vi "AxisGetConfFromFile.vi"(7 "conf file path":path caption="selected path", 8 "error in (no error)":errorcluster, 10 "AxisWriteValuesIn":T3={"AxisTarget"=0.0, "AxisTargetVel"=1.0, "AxisStartReq"=FALSE, "AxisStopReq"=FALSE, "AxisClearReq"=FALSE, "AxisMovetype"=FALSE, "AxisMotorON"=FALSE, "MoveModeControl"=4, "AxisHomingVel"=1.0, "AxisAccDecc"=30.0} {"MoveModeControl" items=["Absolute", "Relative", "Velocity", "Homing"]}, 11 "AxisConfigurationIn":T4={"AxisHomeType"=1, "AxisBacklash"=0.0, "AxisGain"=1.0, "AxisOffset"=0.0, "AxisUnit"=1, "ReqConfRead"=FALSE, "ReqConfWrite"=FALSE, "AxisName"="", "AxisAccDecc"=0.0, "AxisHomeVel"=0.0} {"AxisUnit" items=["mm", "°"]; "AxisHomeType" items=["no homing"=0, "forward limit switch"=1, "backward limit switch"=2, "forward reference"=4, "backward reference"=8]}) -> (0 "error out":errorcluster, 1 "AditionalConfigOut":T2 {"UnitsControl" items=["mm", "°"]}, 2 "AxisWriteValuesOut":T3={"AxisTarget"=0.0, "AxisTargetVel"=1.0, "AxisStartReq"=FALSE, "AxisStopReq"=FALSE, "AxisClearReq"=FALSE, "AxisMovetype"=FALSE, "AxisMotorON"=FALSE, "MoveModeControl"=4, "AxisHomingVel"=1.0, "AxisAccDecc"=30.0} {"MoveModeControl" items=["Absolute", "Relative", "Velocity", "Homing"]}, 3 "AxisConfigurationOut":T4={"AxisHomeType"=1, "AxisBacklash"=0.0, "AxisGain"=1.0, "AxisOffset"=0.0, "AxisUnit"=1, "ReqConfRead"=FALSE, "ReqConfWrite"=FALSE, "AxisName"="", "AxisAccDecc"=0.0, "AxisHomeVel"=0.0} {"AxisUnit" items=["mm", "°"]; "AxisHomeType" items=["no homing"=0, "forward limit switch"=1, "backward limit switch"=2, "forward reference"=4, "backward reference"=8]}, 4 "Comunication":T1={"DeviceIDCtrl"=1, "ProtocolCtrl"=enum."Modbus RTU", "COMportCtrl"="", "IPCtrl"=""})   [LabVIEW 2020, in "SMCD14_lib.lvlib"]
uses:
  SMCD14_lib.lvlib
  AxisConfiguration_typedef.ctl
  AxisWriteValues_typedef.ctl
  <vilib>/Utility/config.llb/Read Key (String).vi
  <vilib>/Utility/config.llb/Read Key (U32).vi
  <vilib>/Utility/config.llb/Read Key (Double).vi
  <vilib>/Utility/config.llb/Read Key (Boolean).vi
  <vilib>/Utility/config.llb/NI_LVConfig.lvlib
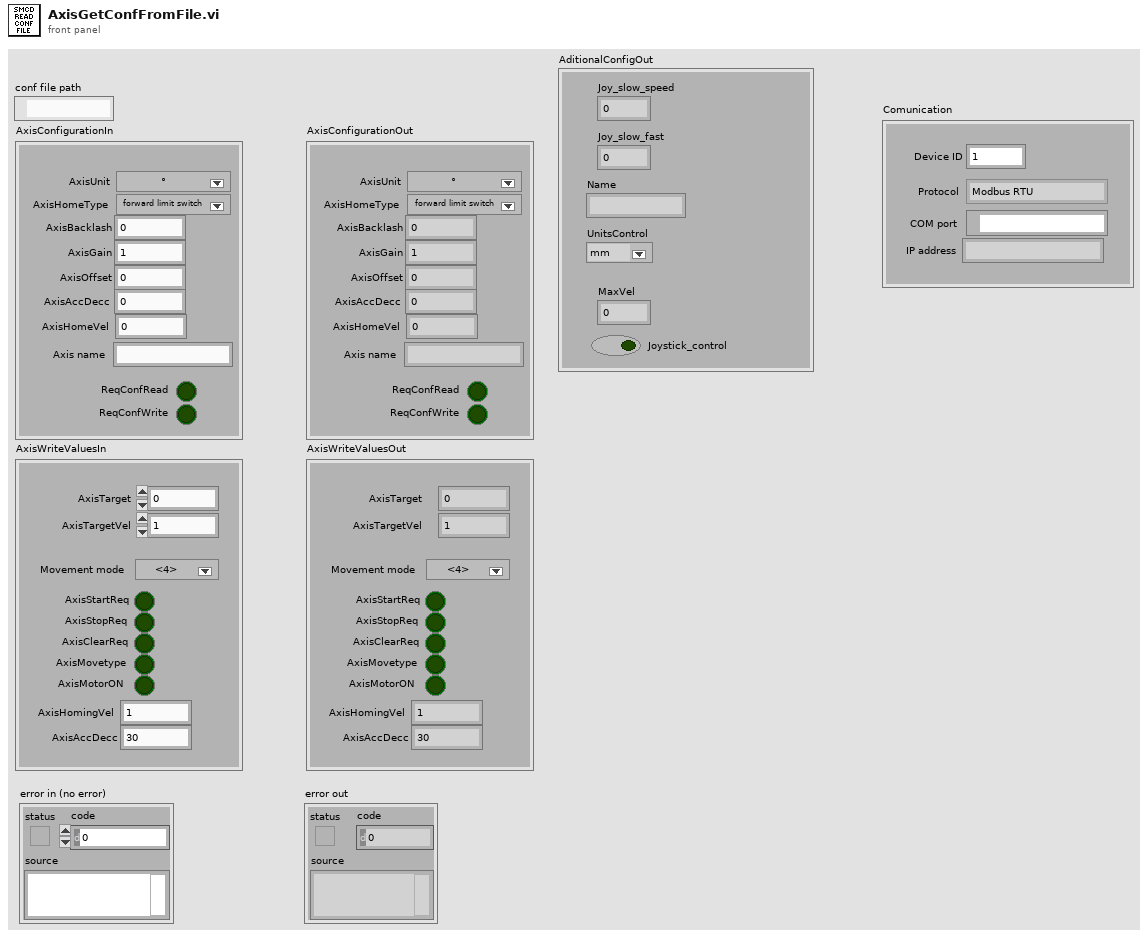
[diagram p1: front panel]
types:
  T1 = cluster{"DeviceIDCtrl":u16, "ProtocolCtrl":enum16{"Modbus RTU", "Modbus TCP", ""}, "COMportCtrl":refnum<visa-resource-name>, "IPCtrl":string}
  T2 = cluster{"Joy_slow_speed":sgl, "Joy_slow_fast":sgl, "Name":string, "UnitsControl":u16, "MaxVel":sgl, "Joystick_control":bool}
  T3 = typedef "SMCD14_lib.lvlib/AxisWriteValues_typedef.ctl" = cluster{"AxisTarget":dbl, "AxisTargetVel":dbl, "AxisStartReq":bool, "AxisStopReq":bool, "AxisClearReq":bool, "AxisMovetype":bool, "AxisMotorON":bool, "MoveModeControl":u16, "AxisHomingVel":dbl, "AxisAccDecc":dbl}
  T4 = typedef "SMCD14_lib.lvlib/AxisConfiguration_typedef.ctl" = cluster{"AxisHomeType":u16, "AxisBacklash":dbl, "AxisGain":dbl, "AxisOffset":dbl, "AxisUnit":u16, "ReqConfRead":bool, "ReqConfWrite":bool, "AxisName":string, "AxisAccDecc":dbl, "AxisHomeVel":dbl}
  T5 = typedef "NI_LVConfig.lvlib/Config Data RefNum.ctl" = refnum<k1>
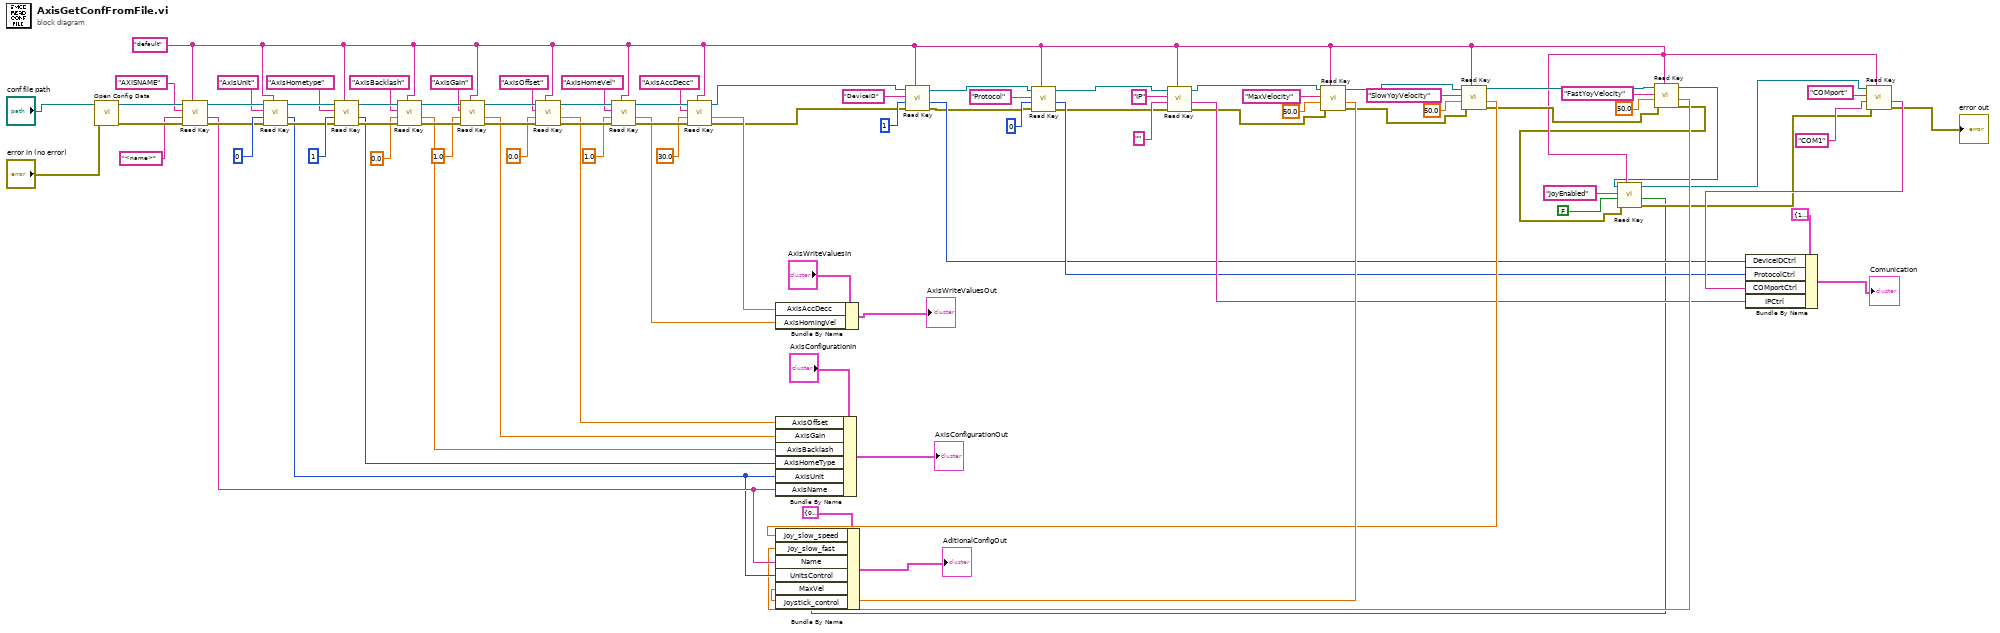
[diagram p0: block diagram]
diagram:
  w8 = "default" ("section")
  n1 = call <vilib>:"Open Config Data.vi"("error in (no error)"="error in (no error)", "configuration file path"="conf file path") -> ("error out"=w91:errorcluster, "refnum"=w92:T5)  [unwired: 7 in, 1 out]
  n2 = call-poly <vilib>:"Read Key.vi"("section"=w8, "error in (no error)"=w91, "default value"="<name>", "key"="AXISNAME", "refnum"=w92) -> ("error out"=w80:errorcluster, "value"=w48:string, "refnum out"=w88:T5)  [unwired: 3 in, 1 out]
  n3 = call-poly <vilib>:"Read Key.vi"("section"=w8, "error in (no error)"=w80, "default value"=u32 0, "key"="AxisUnit", "refnum"=w88) -> ("error out"=w79:errorcluster, "value"=w47:u32, "refnum out"=w85:T5)  [unwired: 3 in, 1 out]
  n4 = call-poly <vilib>:"Read Key.vi"("section"=w8, "error in (no error)"=w79, "default value"=u32 1, "key"="AxisHometype", "refnum"=w85) -> ("error out"=w78:errorcluster, "value"=w58:u32, "refnum out"=w82:T5)  [unwired: 3 in, 1 out]
  n5 = call-poly <vilib>:"Read Key.vi"("section"=w8, "error in (no error)"=w78, "default value"=0.0, "key"="AxisBacklash", "refnum"=w82) -> ("error out"=w75:errorcluster, "value"=w57:dbl, "refnum out"=w76:T5)  [unwired: 3 in, 1 out]
  n6 = call-poly <vilib>:"Read Key.vi"("section"=w8, "error in (no error)"=w75, "default value"=1.0, "key"="AxisGain", "refnum"=w76) -> ("error out"=w71:errorcluster, "value"=w56:dbl, "refnum out"=w72:T5)  [unwired: 3 in, 1 out]
  n7 = call-poly <vilib>:"Read Key.vi"("section"=w8, "error in (no error)"=w71, "default value"=0.0, "key"="AxisOffset", "refnum"=w72) -> ("error out"=w67:errorcluster, "value"=w55:dbl, "refnum out"=w68:T5)  [unwired: 3 in, 1 out]
  n8 = call-poly <vilib>:"Read Key.vi"("section"=w8, "error in (no error)"=w67, "default value"=1.0, "key"="AxisHomeVel", "refnum"=w68) -> ("error out"=w62:errorcluster, "value"=w53:dbl, "refnum out"=w63:T5)  [unwired: 3 in, 1 out]
  n9 = call-poly <vilib>:"Read Key.vi"("section"=w8, "error in (no error)"=w62, "default value"=30.0, "key"="AxisAccDecc", "refnum"=w63) -> ("error out"=w34:errorcluster, "value"=w52:dbl, "refnum out"=w35:T5)  [unwired: 3 in, 1 out]
  n10 = Bundle By Name(cluster="AxisWriteValuesIn", "AxisAccDecc"=w52, "AxisHomingVel"=w53) -> (→"AxisWriteValuesOut":T3)
  n11 = Bundle By Name(cluster="AxisConfigurationIn", "AxisOffset"=w55, "AxisGain"=w56, "AxisBacklash"=w57, "AxisHomeType"=w58, "AxisUnit"=w47, "AxisName"=w48) -> (→"AxisConfigurationOut":T4)
  n12 = call-poly <vilib>:"Read Key.vi"("section"=w8, "error in (no error)"=w34, "default value"=u32 1, "key"="DeviceID", "refnum"=w35) -> ("error out"=w15:errorcluster, "value"=w16:u32, "refnum out"=w44:T5)  [unwired: 3 in, 1 out]
  n13 = call-poly <vilib>:"Read Key.vi"("section"=w8, "error in (no error)"=w15, "default value"=u32 0, "key"="Protocol", "refnum"=w44) -> ("error out"=w14:errorcluster, "value"=w17:u32, "refnum out"=w40:T5)  [unwired: 3 in, 1 out]
  n14 = call-poly <vilib>:"Read Key.vi"("section"=w8, "error in (no error)"=w14, "default value"="" ("key"), "key"="IP", "refnum"=w40) -> ("error out"=w13:errorcluster, "value"=w18:string, "refnum out"=w37:T5)  [unwired: 3 in, 1 out]
  n15 = call-poly <vilib>:"Read Key.vi"("section"=w8, "error in (no error)"=w13, "default value"=50.0, "key"="MaxVelocity", "refnum"=w37) -> ("error out"=w12:errorcluster, "value"=w27:dbl, "refnum out"=w31:T5)  [unwired: 3 in, 1 out]
  n16 = call-poly <vilib>:"Read Key.vi"("section"=w8, "error in (no error)"=w12, "default value"=50.0, "key"="SlowYoyVelocity", "refnum"=w31) -> ("error out"=w11:errorcluster, "value"=w26:dbl, "refnum out"=w28:T5)  [unwired: 3 in, 1 out]
  n17 = call-poly <vilib>:"Read Key.vi"("section"=w8, "error in (no error)"=w11, "default value"=50.0, "key"="FastYoyVelocity", "refnum"=w28) -> ("error out"=w5:errorcluster, "value"=w25:dbl, "refnum out"=w7:T5)  [unwired: 3 in, 1 out]
  n18 = call-poly <vilib>:"Read Key.vi"("section"=w8, "error in (no error)"=w5, "default value"=FALSE, "key"="JoyEnabled", "refnum"=w7) -> ("error out"=w4:errorcluster, "value"=w1:bool, "refnum out"=w6:T5)  [unwired: 3 in, 1 out]
  n19 = Bundle By Name(cluster=T2 {"Joy_slow_speed"=0.0, "Joy_slow_fast"=0.0, "Name"="", "UnitsControl"=0, "MaxVel"=0.0, "Joystick_control"=FALSE} ("JoyControl"), "Joy_slow_speed"=w26, "Joy_slow_fast"=w25, "Name"=w48, "UnitsControl"=w47, "MaxVel"=w27, "Joystick_control"=w1) -> (→"AditionalConfigOut":T2)
  n20 = call-poly <vilib>:"Read Key.vi"("section"=w8, "error in (no error)"=w4, "default value"="COM1", "key"="COMport", "refnum"=w6) -> ("error out"=→"error out":errorcluster, "value"=w19:string)  [unwired: 3 in, 2 out]
  n21 = Bundle By Name(cluster=T1 {"DeviceIDCtrl"=1, "ProtocolCtrl"=enum."Modbus RTU", "COMportCtrl"="", "IPCtrl"=""} ("Comunication 2"), "DeviceIDCtrl"=w16, "ProtocolCtrl"=w17, "COMportCtrl"=w19, "IPCtrl"=w18) -> (→"Comunication":T1)
